vi "_EnqueueMessage.vi"(5 "In Front? (F)":bool, 7 "Timeout (-1 ms)":i32, 8 "error in (no error)":errorcluster, 10 "Message":refnum<class "Message.lvclass">, 11 "MessageQueue":refnum<class "PrefixQueue.lvclass">) -> (0 "error out":errorcluster, 3 "MessageQueue out":refnum<class "PrefixQueue.lvclass">, 4 "Timed Out?":bool)   [LabVIEW 2009, in "LapDog.Messaging.v2.PrefixQueue.lvlib" / "PrefixQueue.lvclass"]
doc: "This protected method the MessageQueue._EnqueueMessage method. This allows users to use the polymorphic EnqueueMessage method on the palette with PrefixQueue objects.\n\nPrepends the prefix to the message name and adds it to the queue. By default the message is added to the rear of the queue. Set 'In Front?' to TRUE to add the message to the front of the queue.\n\nThis method executes regardless of the error in state."
uses:
  PrefixQueue.lvclass
  Messaging.v2/MessageObject/Message.lvclass
  Messaging.v2/MessageQueue/MessageQueue.lvclass
  PrefixQueue.lvclass/PrefixQueue.ctl
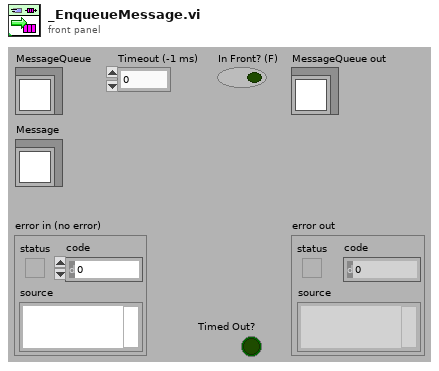
[diagram p1: front panel]
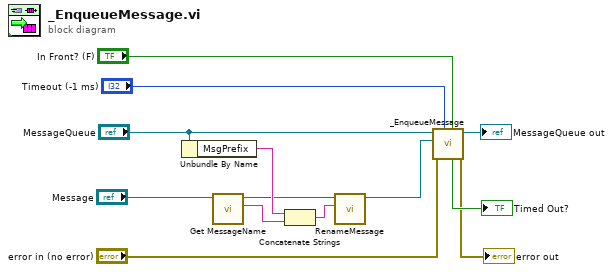
[diagram p0: block diagram]
diagram:
  n1 = Unbundle By Name("MessageQueue") -> ("MsgPrefix"=w11:string)
  n2 = call "Get MessageName.vi"("Message in"="Message") -> ("Message Name"=w3:string, "Message out"=w1:refnum<class "Message.lvclass">)  [unwired: 8 in, 1 out]
  n3 = Concatenate Strings(w11, w3) -> (w2:string)
  n4 = call "RenameMessage.vi"("Message Name"=w2, "Message in"=w1) -> ("Message out"=w4:refnum<class "Message.lvclass">)  [unwired: 8 in, 1 out]
  n5 = call-parent "_EnqueueMessage.vi"("In Front? (F)"="In Front? (F)", "Timeout (-1 ms)"="Timeout (-1 ms)", "error in (no error)"="error in (no error)", "Message"=w4, "MessageQueue"="MessageQueue") -> ("error out"=→"error out":errorcluster, "MessageQueue out"=→"MessageQueue out":refnum<class "PrefixQueue.lvclass">, "Timed Out?"=→"Timed Out?":bool)  [unwired: 4 in]
